vi "Extract-State-from-Array-of-States.vi"(5 "Current State":string, 9 "Array of States to Process":T1[](array[typedef])) -> (8 "Modified Array of States to Process":T1)   [LabVIEW 2016]
uses:
  controls/state control sample changer.ctl
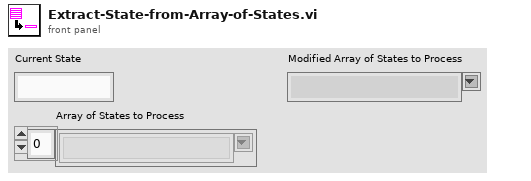
[diagram p1: front panel]
types:
  T1 = typedef "state control sample changer.ctl" = string
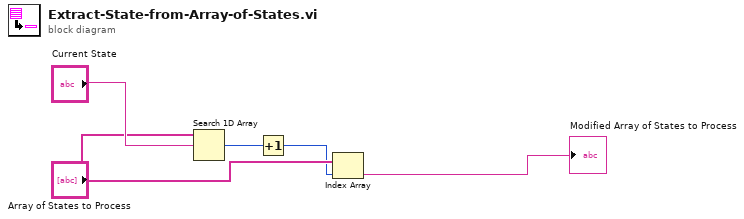
[diagram p0: block diagram]
diagram:
  n1 = Search 1D Array(1D array="Array of States to Process", element="Current State") -> (index of element=w3:i32)  [unwired: 1 in]
  n2 = Increment(x=w3) -> (x+1=w2:i32)
  n3 = Index Array(array="Array of States to Process", index=w2) -> (element=→"Modified Array of States to Process":T1)
